vi "RSZVB Set Renormalization Mode.vi"(8 "error in (no error)":errorcluster {"code" format="%.0x"}, 9 "Mode (Auto)":i32(ring) items=["Auto", "Explicit"], 11 "VISA session":refnum<visa-resource-name>) -> (0 "error out":errorcluster {"code" format="%.0x"}, 3 "dup VISA session":refnum<visa-resource-name>)   [LabVIEW 2011]
doc: "This VI controls the renormalization rules for data export and import globally. \n\nRemote-control command(s):\nMMEMory:SETTings:RENorm:MODE"
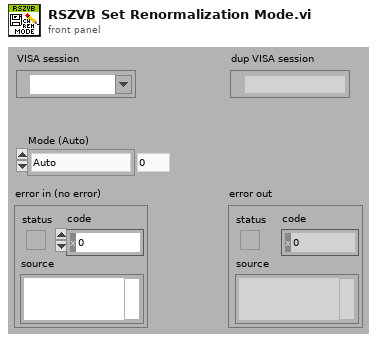
[diagram p1: front panel]
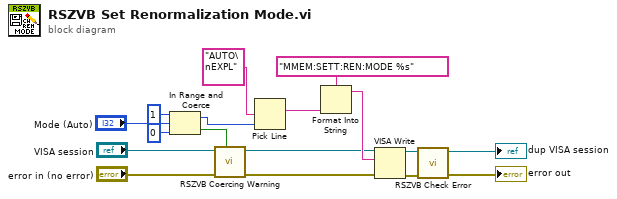
[diagram p0: block diagram]
diagram:
  n1 = In Range and Coerce(upper limit=1, x="Mode (Auto)", lower limit=0) -> (coerced(x)=w1:i32, In Range?=w6:bool)
  n2 = call "RSZVB Coercing Warning.vi"("In Range?"=w6, "error in (no error)"="error in (no error)", "VISA session"="VISA session") -> ("error out"=w2:errorcluster, "dup VISA session"=w3:refnum<visa-resource-name>)  [unwired: 7 in]
  n3 = Pick Line(multi-line string="AUTO\nEXPL", line index=w1) -> (output string=w15:string)  [unwired: 1 in]
  n4 = Format Into String(format string="MMEM:SETT:REN:MODE %s", w15) -> (resulting string=w14:string)  [unwired: 2 in, 1 out]
  n5 = VISA Write(VISA resource name=w3, write buffer=w14, error in (no error)=w2) -> (VISA resource name out=w12:refnum<visa-resource-name>, error out=w13:errorcluster)  [unwired: 1 out]
  n6 = call "RSZVB Check Error.vi"("error in (no error)"=w13, "VISA session"=w12) -> ("error out"=→"error out":errorcluster, "dup VISA session"=→"dup VISA session":refnum<visa-resource-name>)  [unwired: 8 in]
